vi "Get Number.vi"() -> (3 "Number":dbl)   [LabVIEW 2016]
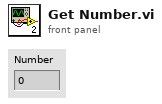
[diagram p1: front panel]
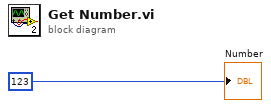
[diagram p0: block diagram]
diagram:
  "Number" <- 123
